vi "Alter Macro V2.vi"(7 "Action":enum16{"Add", "Insert", "Modify", "Delete"}(ring)=enum."Delete", 9 "Step":i32, 11 "Macro":refnum<class "Macro.lvclass">) -> (3 "Macro out":refnum<class "Macro.lvclass">)   [LabVIEW 2020, in "MacroAssert.lvlib"]
doc: "Higher level VI for performing a number of actions on a profile. Takes <B>Action</B> as an input and executes code that performs that action.\n\nThis V2 is meant to be used in conjunction with the double click functionality that was put in as a patch."
uses:
  MacroAssert.lvlib
  Classes/Macro/Macro.lvclass
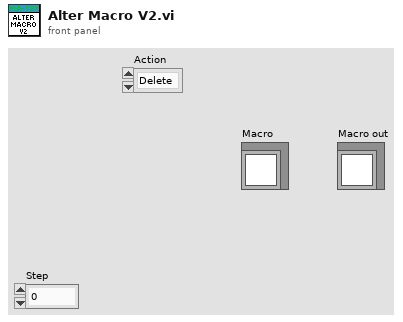
[diagram p1: front panel]
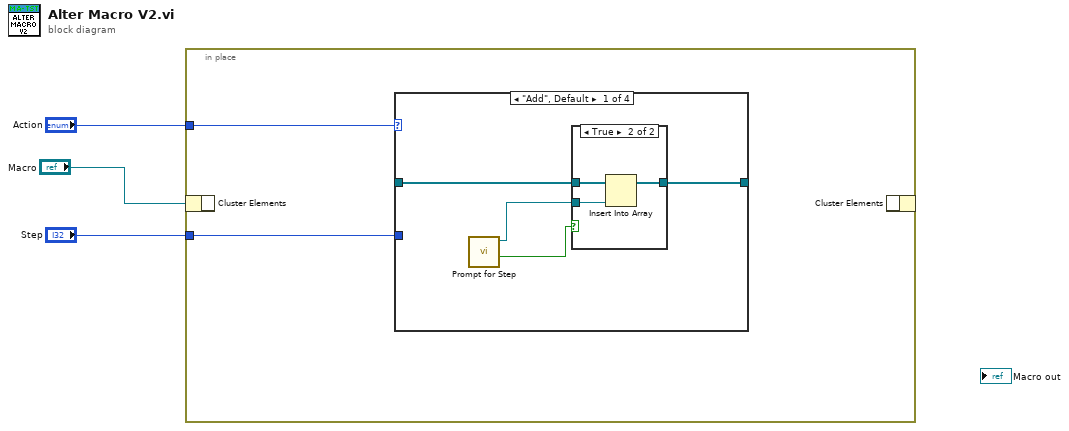
[diagram p0: block diagram]
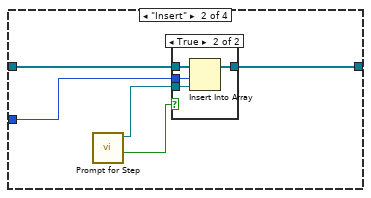
[diagram p3: hidden frame]
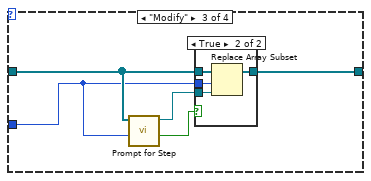
[diagram p5: hidden frame]
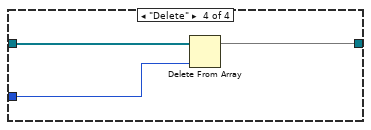
[diagram p7: hidden frame]
diagram:
  n1 = in-place {
    in-place-border: "Action" -> [w7]
    in-place-border: "Step" -> [w6]
    n2 = in-place-cluster #1("Macro") -> ()  [unwired: 1 out]
    n3 = case shown="\"Add\", Default" w7 {
      tunnel: [w8 w20 w30 w38] -> w4
      tunnel: [w10 w19 w29 w37] -> w5
      tunnel: w6 -> [_ w16 w27 w36]
      frame "Add", Default {
        n4 = call "Prompt for Step.vi"() -> ("OK?"=w9:bool, "Step"=w11:refnum<class "Step.lvclass">)  [unwired: 9 in, 1 out]
        n5 = case shown="True" w9 {
          tunnel: w11 -> [_ w15]
          tunnel: w8 -> [w12 w14]
          tunnel: [w12 w13] -> w10
          frame False {
          }
          frame True {
            n6 = Insert Into Array(array=w14, new element=w15) -> (w13:refnum<class "Step.lvclass">[])  [unwired: 1 in]
          }
        }
      }
      frame "Insert" {
        n7 = call "Prompt for Step.vi"() -> ("OK?"=w17:bool, "Step"=w18:refnum<class "Step.lvclass">)  [unwired: 9 in, 1 out]
        n8 = case shown="True" w17 {
          tunnel: w16 -> [_ w25]
          tunnel: w18 -> [_ w24]
          tunnel: w20 -> [w21 w23]
          tunnel: [w21 w22] -> w19
          frame False {
          }
          frame True {
            n9 = Insert Into Array(array=w23, index=w25, new element=w24) -> (w22:refnum<class "Step.lvclass">[])
          }
        }
      }
      frame "Modify" {
        n10 = call "Prompt for Step.vi"("Index"=w27, "Steps"=w30) -> ("OK?"=w28:bool, "Step"=w26:refnum<class "Step.lvclass">)  [unwired: 7 in, 1 out]
        n11 = case shown="True" w28 {
          tunnel: w27 -> [_ w35]
          tunnel: w26 -> [_ w34]
          tunnel: [w31 w33] -> w29
          tunnel: w30 -> [w31 w32]
          frame False {
          }
          frame True {
            n12 = Replace Array Subset(array=w32, new element=w34, index=w35) -> (w33:refnum<class "Step.lvclass">[])
          }
        }
      }
      frame "Delete" {
        n13 = Delete From Array(array=w38, index=w36) -> (array with subset deleted=w37)  [unwired: 1 in, 1 out]
      }
    }
    n14 = in-place-cluster #1() -> ()  [unwired: 1 in, 1 out]
  }
